vi "XY Graph Add Multiplots with Names.vi"(0 "XYGraph in":T3, 1 "Array of Scales (Default)":cluster{"X Scale":u32, "Y Scale":u32}[](array[cluster]), 2 "Plots Interpolation (Previous Plot's Style)":T2[](array[typedef]) items=["Point (.)", "Stepwise Right (--.)", "Line + Point (\\. /)", "Stepwise Left (.--)", "Stepwise Centered (-.-)", "Stepwise Vertical (|.|)", "Line (-)", "Use Previous Plot's Style"], 3 "Keep Existing Plots (T)":bool=TRUE, 5 "Array of Plots":cluster{"X Array":dbl[], "Y Array":dbl[]}[](array[cluster]), 7 "Plots Metadata":variant[](array[variant]), 9 "Array of Plot Names (\"Plot\")":string[](array[string]), 11 "error in (no error)":errorcluster, 12 "Make Visible (T)":bool=TRUE, 13 "Plot Colors (Default)":u32[](array[colorbox]), 14 "Point Style (Dot)":T1=enum."Dot") -> (4 "XY Graph Caption (or Label)":string, 6 "Total Number of Plots":i32, 8 "Number of Plots Added":i32, 10 "Added Plot Names":string[](array[string]), 15 "error out":errorcluster)   [LabVIEW 2021, in "XY Graph Add-Ons.lvlib"]
uses:
  XY Graph Add-Ons.lvlib
  XY Graph Refnum.ctl
  LabVIEW Plot Interpolation.ctl
  Plot Point Style.ctl
  XY Graph Get Plots Metadata.vi
  XY Graph Set Plots Metadata.vi
  Strings/Strings.lvlib
  Graphs.lvlib
  Error/Error.lvlib
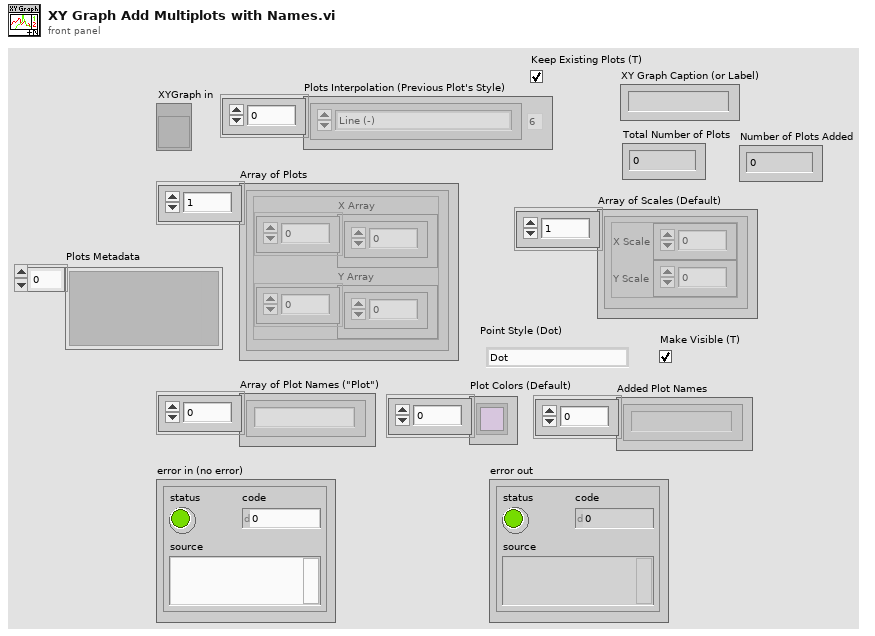
[diagram p1: front panel]
types:
  T1 = typedef "Graphs.lvlib/Plot Point Style.ctl" = enum16{"not defined", "None", "Empty Circle", "Filled Circle", "Thick Circle", "Dotted Circle", "Empty Square", "Filled Square", "Thick Square", "Dotted Square", "Small Filled Square", "Dot", "Cross", "Tiny Cross", "Large X", "Small x", "Diamond", "Small Empty Square"}
  T2 = typedef "Graphs.lvlib/LabVIEW Plot Interpolation.ctl" = u8
  T3 = typedef "XY Graph Add-Ons.lvlib/XY Graph Refnum.ctl" = refnum<vi>
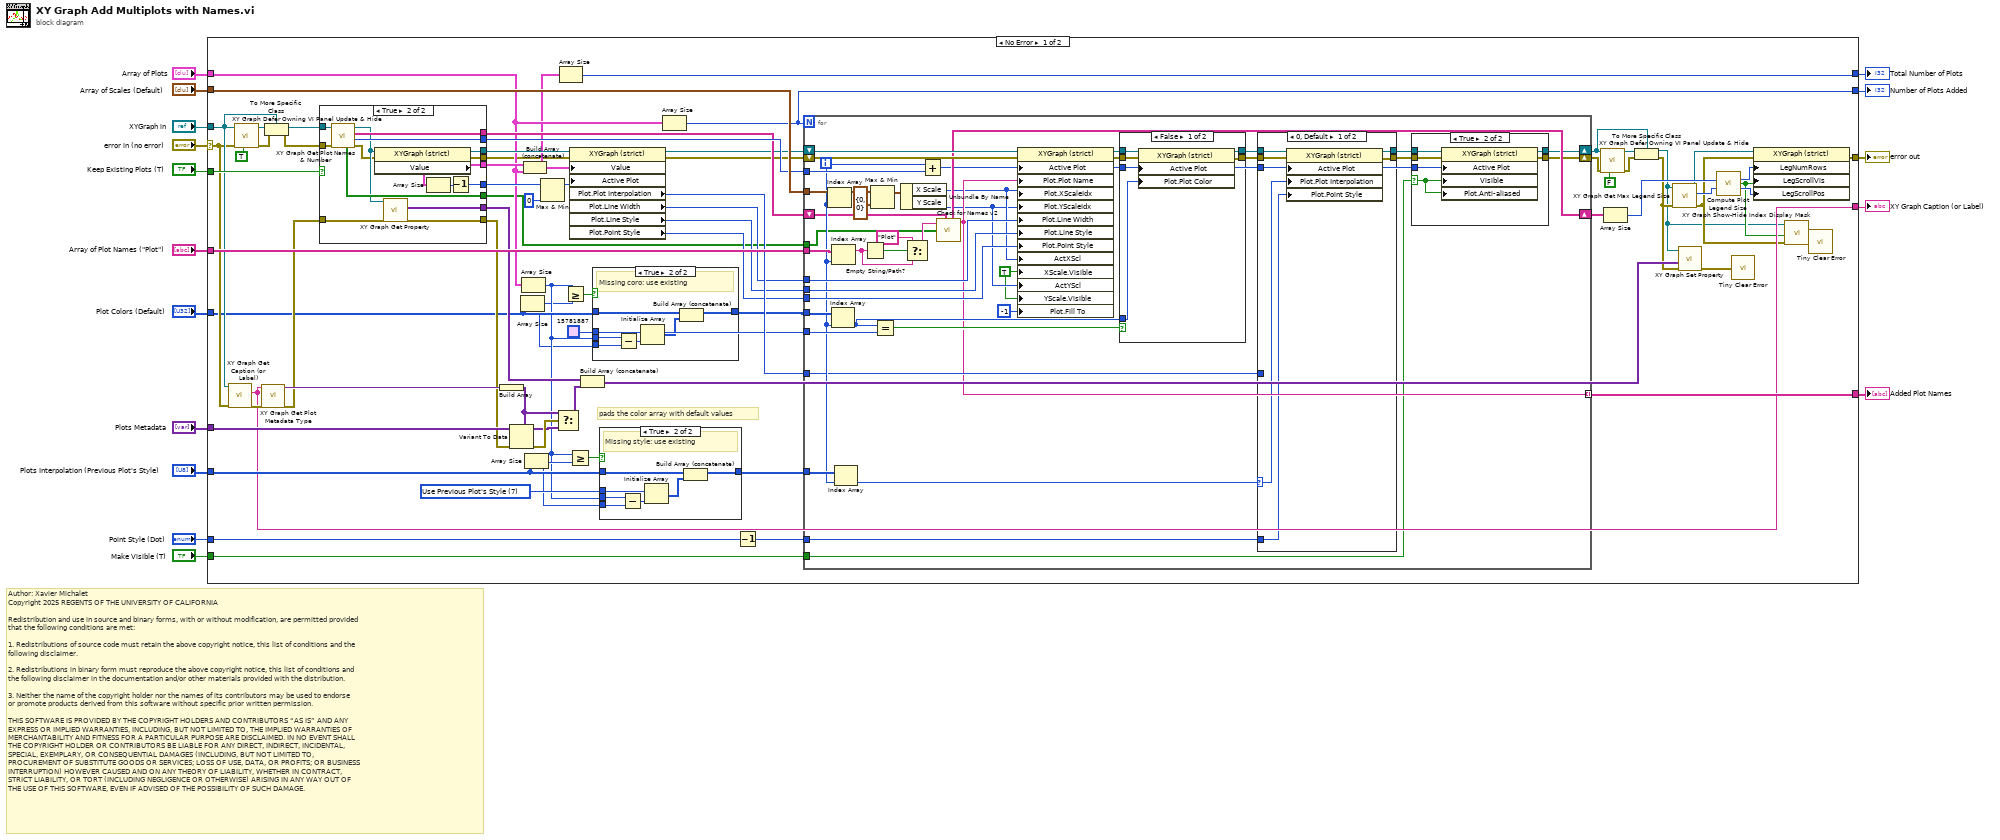
[diagram p0: block diagram]
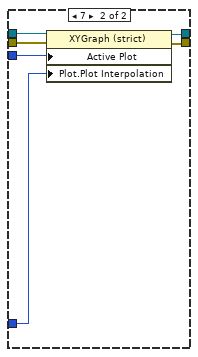
[diagram p4: hidden frame]
diagram:
  # "Author: Xavier Michalet\nCopyright 2025 REGENTS OF THE UNIVERSITY OF CALIFORNIA\n\nRedistribution and use in source and binary forms, with or without modification, are permitted provided\nthat the following conditions are met:\n\n1. Redistributions of source code must retain the above copyright notice, this list of conditions and the\nfollowing disclaimer.\n\n2. Redistributions in binary form must reproduce the above copyright notice, this list of conditions and\nthe following disclaimer in the documentation and/or other materials provided with the distribution.\n\n3. Neither the name of the copyright holder nor the names of its contributors may be used to endorse \nor promote products derived from this software without specific prior written permission.\n\nTHIS SOFTWARE IS PROVIDED BY THE COPYRIGHT HOLDERS AND CONTRIBUTORS “AS IS” AND ANY \nEXPRESS OR IMPLIED WARRANTIES, INCLUDING, BUT NOT LIMITED TO, THE IMPLIED WARRANTIES OF\nMERCHANTABILITY AND FITNESS FOR A PARTICULAR PURPOSE ARE DISCLAIMED. IN NO EVENT SHALL\nTHE COPYRIGHT HOLDER OR CONTRIBUTORS BE LIABLE FOR ANY DIRECT, INDIRECT, INCIDENTAL, \nSPECIAL, EXEMPLARY, OR CONSEQUENTIAL DAMAGES (INCLUDING, BUT NOT LIMITED TO, \nPROCUREMENT OF SUBSTITUTE GOODS OR SERVICES; LOSS OF USE, DATA, OR PROFITS; OR BUSINESS\nINTERRUPTION) HOWEVER CAUSED AND ON ANY THEORY OF LIABILITY, WHETHER IN CONTRACT, \nSTRICT LIABILITY, OR TORT (INCLUDING NEGLIGENCE OR OTHERWISE) ARISING IN ANY WAY OUT OF\nTHE USE OF THIS SOFTWARE, EVEN IF ADVISED OF THE POSSIBILITY OF SUCH DAMAGE."
  n1 = case shown="No Error" "error in (no error)" {
    selector: "error in (no error)" -> [w31 w196]
    tunnel: "XYGraph in" -> [w41 _]
    tunnel: "Array of Plot Names (\"Plot\")" -> [w88 _]
    tunnel: "Array of Scales (Default)" -> [w87 _]
    tunnel: [w78 _] -> w12
    tunnel: "Array of Plots" -> [w77 _]
    tunnel: "Plot Colors (Default)" -> [w21 _]
    tunnel: "Plots Interpolation (Previous Plot's Style)" -> [w76 _]
    tunnel: "Keep Existing Plots (T)" -> [w71 _]
    tunnel: [w70 w196] -> w7
    tunnel: [w68 _] -> w6
    tunnel: "Point Style (Dot)" -> [w67 _]
    tunnel: "Make Visible (T)" -> [w65 _]
    tunnel: [w63 _] -> w3
    tunnel: [w29 _] -> w2
    tunnel: "Plots Metadata" -> [w39 _]
    frame No Error {
      w74 = T2 7 items=["Point (.)", "Stepwise Right (--.)", "Line + Point (\\. /)", "Stepwise Left (.--)", "Stepwise Centered (-.-)", "Stepwise Vertical (|.|)", "Line (-)", "Use Previous Plot's Style"] ("Plot Interpolation")
      w19 = u32 15781887 ("Plot Color (Default)")
      # "pads the color array with default values"
      n2 = call "XY Graph Get Caption (or Label).vi"("error in (no error)"=w31, "XY Graph in"=w41) -> ("error out"=w30:errorcluster, "Caption (or Label) Text"=w29:string)  [unwired: 7 in, 1 out]
      n3 = call "XY Graph Defer Owning VI Panel Update & Hide.vi"("Defer Owning Panel Update"=TRUE, "error in (no error)"=w31, "XY Graph Refnum in"=w41) -> ("error out"=w54:errorcluster, "XY Graph Refnum out"=w57:refnum<vi>)  [unwired: 7 in]
      n4 = call "XY Graph Get Plot Metadata Type.vi"("Error In"=w30, "Graph Label"=w29) -> ("Error Out"=w34:errorcluster, "Plot Metadata Type"=w40:variant)  [unwired: 7 in, 1 out]
      n5 = To More Specific Class(target class=w41, reference=w57, error in=w54) -> (specific class reference=w55:T3, error out=w53:errorcluster)
      n6 = case shown="True" w71 {
        tunnel: [w172 w187] -> w89
        tunnel: w55 -> [w172 w186]
        tunnel: w53 -> [w171 w185]
        tunnel: [_ w184] -> w86
        tunnel: [_ w182] -> w85
        tunnel: [_ w181] -> w84
        tunnel: [_ w180] -> w83
        tunnel: [w171 w179] -> w64
        tunnel: [_ w178] -> w56
        tunnel: [_ w176] -> w44
        tunnel: w34 -> [w170 w174]
        tunnel: [w170 w173] -> w33
        frame False {
        }
        frame True {
          n7 = call "XY Graph Get Plot Names & Number.vi"("error in (no error)"=w185, "XYGraph in"=w186) -> ("error out"=w175:errorcluster, "# Plots"=w181:i32, "Plot Names"=w180:string[], "XYGraph out"=w177:T3, "Empty Plots?"=w178:bool[])  [unwired: 4 in, 1 out]
          n8 = property class="XYGraph (strict)"(reference=w177, error in=w175) -> (reference out=w187:T3, error out=w179:errorcluster, "Value"=w184:cluster{"X Array":dbl[], "Y Array":dbl[]}[])
          n9 = call-poly "XY Graph Get Property.vi"("Error In"=w174, "XYGraph Ref"=w177) -> ("Error Out"=w173:errorcluster, "Plot Metadata"=w176:variant[])  [unwired: 6 in, 2 out]
          n10 = Array Size(array=w184) -> (size(s)=w183:i32)
          n11 = Decrement(x=w183) -> (x-1=w182:i32)
        }
      }
      n12 = Build Array(w40) -> (w36:variant[])
      n13 = Variant To Data(error in=w33, type=w36, Variant=w39) -> (data=w37:variant[], error out=w38:errorcluster)
      n14 = Array Size(array=w21) -> (size(s)=w17:i32)
      n15 = Array Size(array=w77) -> (size(s)=w18:i32)
      n16 = Build Array (concatenate)(w86, w77) -> (w69:cluster{"X Array":dbl[], "Y Array":dbl[]}[])
      n17 = Array Size(array=w76) -> (size(s)=w23:i32)
      n18 = Max & Min(x=w85, y=0) -> (max(x,y)=w73:i32)  [unwired: 1 out]
      n19 = Select(t=w36, s=w38, f=w37) -> (s? t:f=w35:variant[])
      n20 = Array Size(array=w69) -> (size(s)=w68:i32)
      n21 = Greater Or Equal?(x=w18, y=w17) -> (x >= y?=w22:bool)
      n22 = Greater Or Equal?(x=w18, y=w23) -> (x >= y?=w24:bool)
      n23 = property class="XYGraph (strict)"(reference=w89, error in=w64, "Value"=w69, "Active Plot"=w73) -> (reference out=w62:T3, error out=w61:errorcluster, "Plot.Plot Interpolation"=w82:u8, "Plot.Line Width"=w81:u8, "Plot.Line Style"=w80:u8, "Plot.Point Style"=w79:u8)
      n24 = Build Array (concatenate)(w44, w35) -> (w43:variant[])
      n25 = case shown="True" w22 {
        tunnel: w21 -> [w91 w98]
        tunnel: [w91 w97] -> w20
        tunnel: w19 -> [_ w95]
        tunnel: w18 -> [_ w94]
        tunnel: w17 -> [_ w93]
        frame False {
        }
        frame True {
          # "Missing coro: use existing"
          n26 = Subtract(x=w94, y=w93) -> (x-y=w96:i32)
          n27 = Initialize Array(w95, w96) -> (w92:u32[])
          n28 = Build Array (concatenate)(w98, w92) -> (w97:u32[])
        }
      }
      n29 = case shown="True" w24 {
        tunnel: w76 -> [w188 w195]
        tunnel: [w188 w194] -> w75
        tunnel: w74 -> [_ w192]
        tunnel: w18 -> [_ w191]
        tunnel: w23 -> [_ w190]
        frame False {
        }
        frame True {
          # "Missing style: use existing"
          n30 = Subtract(x=w191, y=w190) -> (x-y=w189:i32)
          n31 = Initialize Array(w192, w189) -> (w193:T2[])
          n32 = Build Array (concatenate)(w195, w193) -> (w194:T2[])
        }
      }
      n33 = Array Size(array=w77) -> (size(s)=w63:i32)
      n34 = Decrement(x=w67) -> (x-1=w66:T1)
      n35 = for {
        N: w63 -> [_]
        tunnel: w88 -> [w137]
        shift-right: [w107] -> w60
        shift-left: w61 -> [w139]
        shift-right: [w110] -> w46
        shift-left: w62 -> [w140]
        tunnel: w84 -> [w138]
        shift-right: [w113] -> w90
        shift-left: w83 -> [w114]
        tunnel: w87 -> [w136]
        tunnel: w82 -> [w116]
        tunnel: w81 -> [w131]
        tunnel: w80 -> [w130]
        tunnel: w79 -> [w129]
        tunnel: [w111] -> w78 mode=indexing
        tunnel: w20 -> [w128]
        tunnel: w19 -> [w127]
        tunnel: w75 -> [w119]
        tunnel: w66 -> [w115]
        tunnel: w65 -> [w109]
        tunnel: w56 -> [w103]
        i -> [w118]
        w100 = TRUE ("X Scale.Visible")
        n36 = Index Array(array=w136, index=w118) -> (element=w135:cluster{"X Scale":u32, "Y Scale":u32})
        n37 = Index Array(array=w128, index=w118) -> (element=w123:u32)
        n38 = Index Array(array=w137, index=w118) -> (element=w133:string)
        n39 = Index Array(array=w119, index=w118) -> (element=w117:T2)
        n40 = Empty String/Path?(string/path=w133) -> (empty?=w134:bool)
        n41 = Max & Min(x=w135, y=cluster{"X Scale":u32, "Y Scale":u32} {"X Scale"=0, "Y Scale"=0}) -> (max(x,y)=w105:cluster{"X Scale":u32, "Y Scale":u32})  [unwired: 1 out]
        n42 = Equal?(x=w123, y=w127) -> (x = y?=w126:bool)
        n43 = Unbundle By Name(w105) -> ("X Scale"=w102:u32, "Y Scale"=w101:u32)
        n44 = Select(t="Plot", s=w134, f=w133) -> (s? t:f=w112:string)
        n45 = Add(x=w118, y=w138) -> (x+y=w106:i32)
        n46 = call "Check for Names v2.vi"("New Name"=w112, "Name List"=w114, "Empty Plots?"=w103) -> ("New Name List"=w113:string[], "New Name"=w111:string)  [unwired: 3 in, 2 out]
        n47 = property class="XYGraph (strict)"(reference=w140, error in=w139, "Active Plot"=w106, "Plot.Plot Name"=w111, "Plot.XScaleIdx"=w102, "Plot.YScaleIdx"=w101, "Plot.Line Width"=w131, "Plot.Line Style"=w130, "Plot.Point Style"=w129, "ActXScl"=w102, "XScale.Visible"=w100, "ActYScl"=w101, "YScale.Visible"=w100, "Plot.Fill To"=i16 -1) -> (reference out=w125:T3, error out=w124:errorcluster)
        n48 = case shown="False" w126 {
          tunnel: w125 -> [w167 w169]
          tunnel: [w166 w169] -> w122
          tunnel: w124 -> [w165 w168]
          tunnel: [w164 w168] -> w121
          tunnel: w123 -> [w163 _]
          tunnel: w106 -> [w162 _]
          frame False {
            n49 = property class="XYGraph (strict)"(reference=w167, error in=w165, "Active Plot"=w162, "Plot.Plot Color"=w163) -> (reference out=w166:T3, error out=w164:errorcluster)
          }
          frame True {
          }
        }
        n50 = case shown="0, Default" w117 {
          selector: w117 -> [w150 _]
          tunnel: w122 -> [w155 w161]
          tunnel: [w154 w160] -> w120
          tunnel: w121 -> [w153 w159]
          tunnel: [w152 w158] -> w108
          tunnel: w106 -> [w151 w157]
          tunnel: w116 -> [_ w156]
          tunnel: w115 -> [w149 _]
          frame 0, Default {
            n51 = property class="XYGraph (strict)"(reference=w155, error in=w153, "Active Plot"=w151, "Plot.Plot Interpolation"=w150, "Plot.Point Style"=w149) -> (reference out=w154:T3, error out=w152:errorcluster)
          }
          frame 7 {
            n52 = property class="XYGraph (strict)"(reference=w161, error in=w159, "Active Plot"=w157, "Plot.Plot Interpolation"=w156) -> (reference out=w160:T3, error out=w158:errorcluster)
          }
        }
        n53 = case shown="True" w109 {
          selector: w109 -> [_ w143]
          tunnel: w120 -> [w142 w148]
          tunnel: [w142 w147] -> w110
          tunnel: w108 -> [w141 w146]
          tunnel: [w141 w145] -> w107
          tunnel: w106 -> [_ w144]
          frame False {
          }
          frame True {
            n54 = property class="XYGraph (strict)"(reference=w148, error in=w146, "Active Plot"=w144, "Visible"=w143, "Plot.Anti-aliased"=w143) -> (reference out=w147:T3, error out=w145:errorcluster)
          }
        }
      }
      n55 = call "XY Graph Defer Owning VI Panel Update & Hide.vi"("Defer Owning Panel Update"=FALSE, "error in (no error)"=w60, "XY Graph Refnum in"=w46) -> ("error out"=w48:errorcluster, "XY Graph Refnum out"=w47:refnum<vi>)  [unwired: 7 in]
      n56 = Array Size(array=w90) -> (size(s)=w51:i32)
      n57 = To More Specific Class(target class=w46, reference=w47, error in=w48) -> (specific class reference=w25:T3, error out=w42:errorcluster)
      n58 = call "XY Graph Get Max Legend Size.vi"("Error In"=w42, "XYGraph Refnum"=w25) -> ("Error Out"=w27:errorcluster, "Max Legend Size"=w52:i32, "XYGraph Refnum"=w45:T3)  [unwired: 6 in, 1 out]
      n59 = call-poly "XY Graph Set Property.vi"("error in (no error)"=w42, "Plots Metadata"=w43, "XY Graph Refnum"=w25) -> ("error out"=w32:errorcluster)  [unwired: 7 in, 1 out]
      n60 = call "Compute Plot Legend Size.vi"("# Plots"=w51, "Max Legend Size"=w52) -> ("LegNumRows"=w50:u32, "LegScrollVis"=w26:bool, "LegScrollPos"=w49:u32)  [unwired: 11 in]
      n61 = call "Tiny Clear Error.vi"("Error In"=w32) -> ()  [unwired: 8 in, 1 out]
      n62 = property class="XYGraph (strict)"(reference=w45, error in=w27, "LegNumRows"=w50, "LegScrollVis"=w26, "LegScrollPos"=w49) -> (error out=w70:errorcluster)  [unwired: 1 out]
      n63 = call "XY Graph Show-Hide Index Display Mask.vi"("error in (no error)"=w27, "Show(T)/Hide(F)"=w26, "XYGraph Ref"=w25) -> ("error out"=w28:errorcluster)  [unwired: 7 in, 1 out]
      n64 = call "Tiny Clear Error.vi"("Error In"=w28) -> ()  [unwired: 8 in, 1 out]
    }
    frame Error {
    }
  }
  "error out" <- w7
  "Added Plot Names" <- w12
  "Total Number of Plots" <- w6
  "Number of Plots Added" <- w3
  "XY Graph Caption (or Label)" <- w2
